vi "FTW-JSON-SerializeAndDestroy.vi"(0 "JSON":refnum<class "FTW-Container.lvclass">, 9 "Pretty Print":bool, 11 "error in":errorcluster) -> (6 "JSON String (UTF-8)":string, 15 "error out":errorcluster)   [LabVIEW 2015]
uses:
  container/FTW-Container.lvclass
panel:
  # "Inputs"
  # "Outputs"
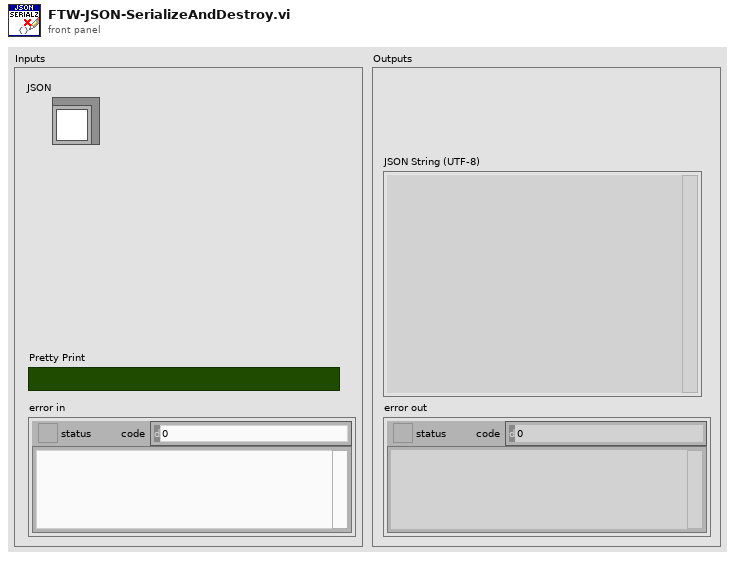
[diagram p1: front panel]
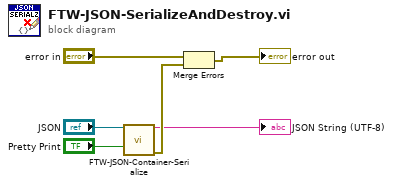
[diagram p0: block diagram]
diagram:
  n1 = call "FTW-JSON-Container-Serialize.vi"("Container"="JSON", "Pretty Print"="Pretty Print") -> ("JSON String"=→"JSON String (UTF-8)":string, "error out"=w3:errorcluster)  [unwired: 12 in]
  n2 = Merge Errors("error in", w3) -> (→"error out":errorcluster)
